vi "NF WF1973_74 QUES Even.vi"(8 "error in (no error)":errorcluster caption="Error IN", 11 "VISAsession":refnum<visa-resource-name>) -> (0 "error out":errorcluster caption="Error OUT", 2 "Query Q_Event":i32=999, 3 "CopyVISAsession":refnum<visa-resource-name>)   [LabVIEW 2010]
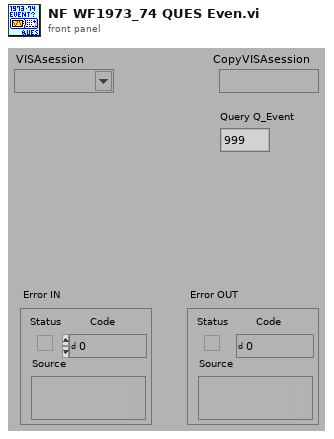
[diagram p1: front panel]
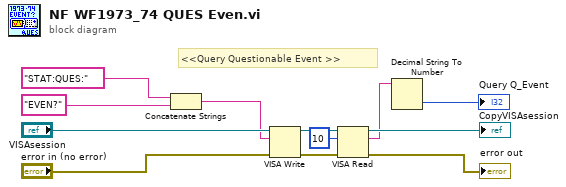
[diagram p0: block diagram]
diagram:
  # "<<Query Questionable Event >>"
  n1 = Concatenate Strings("STAT:QUES:" ("文字列"), "EVEN?" ("文字列")) -> (w1:string)
  n2 = VISA Write(VISA resource name="VISAsession", write buffer=w1, error in (no error)="error in (no error)") -> (VISA resource name out=w4:refnum<visa-resource-name>, error out=w5:errorcluster)  [unwired: 1 out]
  n3 = VISA Read(VISA resource name=w4, byte count=u32 10 ("バイトカウント（0）"), error in (no error)=w5) -> (VISA resource name out=→"CopyVISAsession":refnum<visa-resource-name>, read buffer=w2:string, error out=→"error out":errorcluster)  [unwired: 1 out]
  n4 = Decimal String To Number(string=w2) -> (number=→"Query Q_Event":i32)  [unwired: 2 in, 1 out]
